vi "test_API_rt.vi"() -> ()   [LabVIEW 2014]
uses:
  MQTT.lvlib
  message acknowledgement.ctl
  MQTT client.lvclass
  QoS levels.ctl
panel:
  in  "connect":bool
  out "subid":i32
  in  "subscribe to":string
  in  "subscribe":bool
  in  "QoS":T1=enum."At least once"
  out "send ID":i32
  out "sub_data":string
  out "sub_topic":string
  out "sub_ID":i32
  out "send failure":T2
  out "send success":T2
  out "QOS Ack":T2
  out "disconnected_message":string
  out "disconnected_code":i32
  out "connCode":i32
  out "connected":string
  in  "stop":bool
  in  "send":bool
  in  "data":string
  in  "topic":string
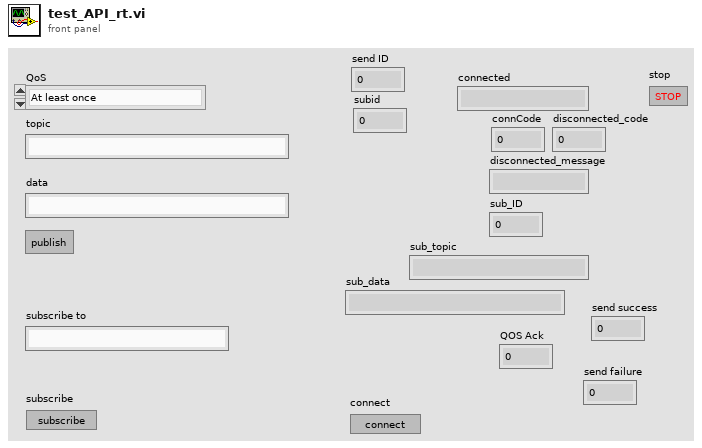
[diagram p1: front panel]
types:
  T1 = typedef "MQTT client.lvclass/QoS levels.ctl" = enum8{"None", "At least once", "Exactly once"}
  T2 = typedef "MQTT client.lvclass/message acknowledgement.ctl" = i32
  T3 = typedef "MQTT.lvlib/events.ctl" = cluster{"subscription":refnum<user-event>, "disconnect":refnum<user-event>, "QoS Ack":refnum<user-event>, "connected":refnum<user-event>, "failed to connect":refnum<user-event>, "send success":refnum<user-event>, "send failure":refnum<user-event>}
  T4 = typedef "MQTT.lvlib/msgAck.ctl" = i32
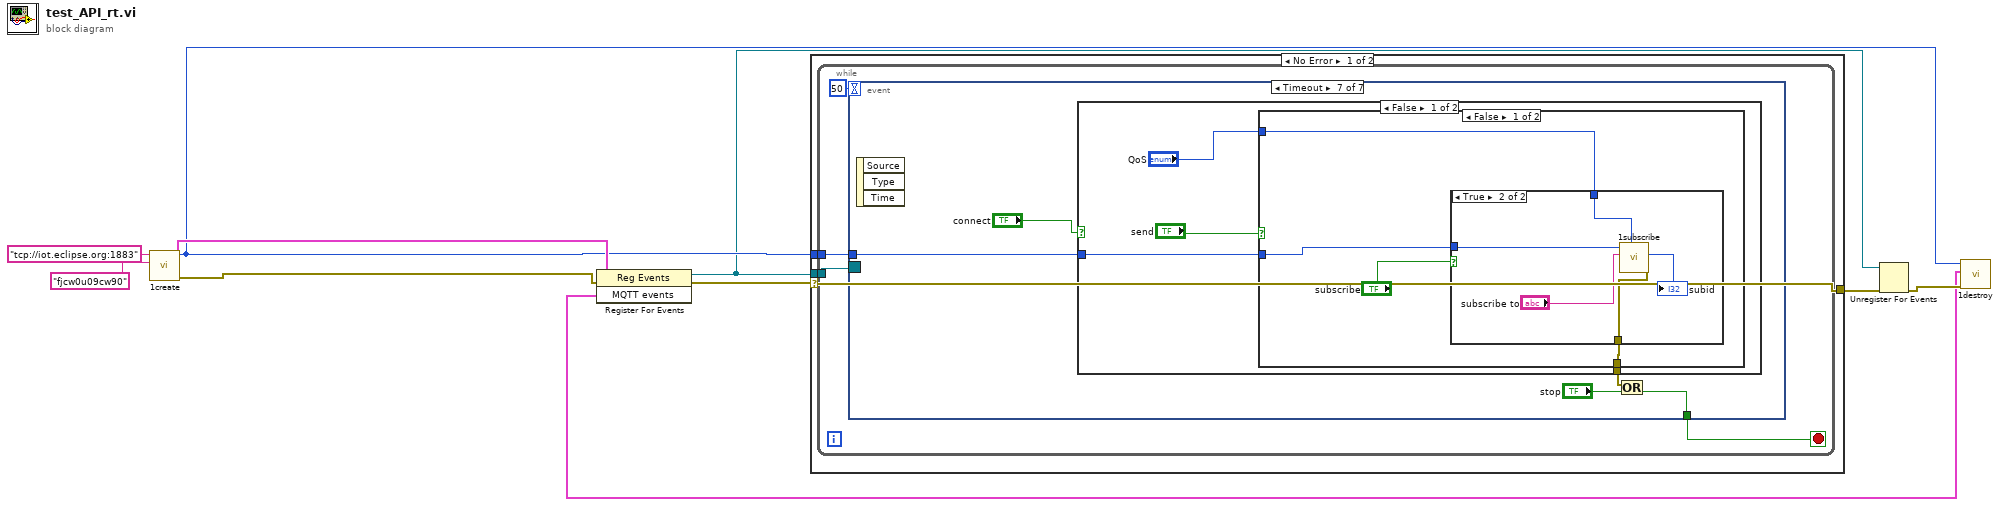
[diagram p0: block diagram]
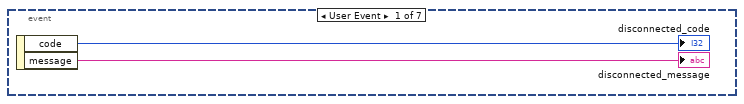
[diagram p2: hidden frame]
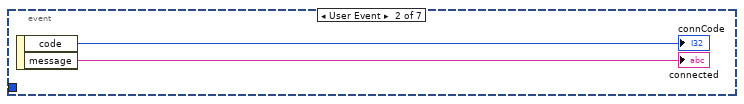
[diagram p3: hidden frame]
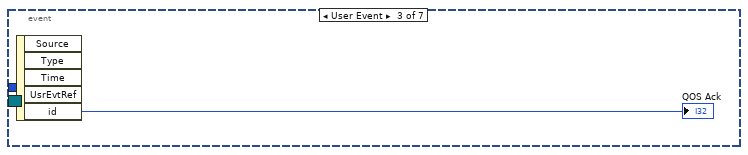
[diagram p4: hidden frame]
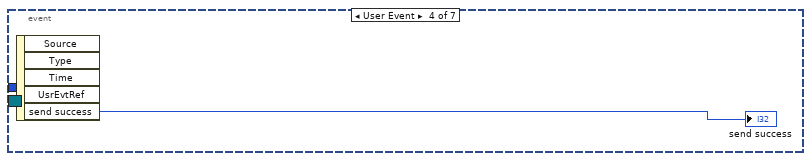
[diagram p5: hidden frame]
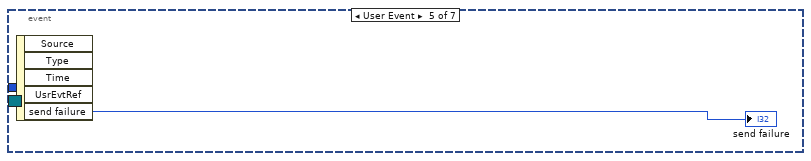
[diagram p6: hidden frame]
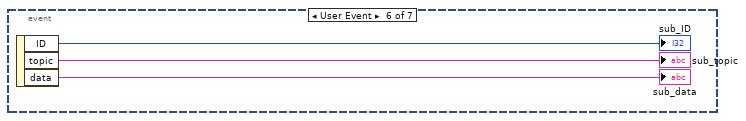
[diagram p7: hidden frame]
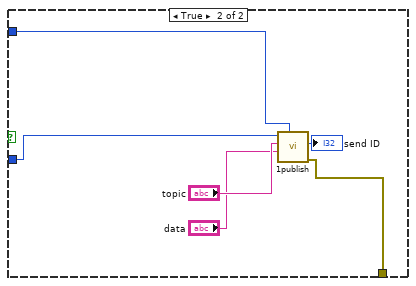
[diagram p9: hidden frame]
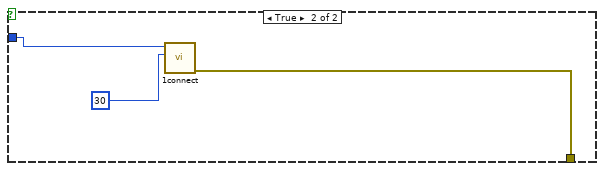
[diagram p10: hidden frame]
diagram:
  n1 = call "1create.vi"("client"="fjcw0u09cw90", "URI"="tcp://iot.eclipse.org:1883") -> ("error out"=w9:errorcluster, "MQTT events"=w3:T3, "MQTT Context"=w2:u64)  [unwired: 7 in]
  n2 = register-events(error in=w9, w3) -> (reference out=w1:refnum<event-registration>, error out=w6:errorcluster)  [unwired: 1 in]
  n3 = case shown="No Error" w6 {
    selector: w6 -> [w10 w54]
    tunnel: w1 -> [w12 _]
    tunnel: [w10 w54] -> w5
    tunnel: w2 -> [w11 _]
    frame No Error {
      n4 = while {
        tunnel: w12 -> [w16]
        tunnel: w11 -> [w15]
        stop <- w14 stop-if-true
        n5 = event shown="[6] Timeout" {
          selector: w16 -> [_ _ _ _ _ _ _]
          dyn-events: _ -> [_ _ _ _ _ _ _]
          timeout: 50 -> [_ _ _ _ _ _ _]
          tunnel: w15 -> [_ _ _ _ _ _ w30]
          tunnel: [_ _ _ _ _ _ w29] -> w14
          event User Event {
            n6 = event-data() -> ("code"=→"disconnected_code":i32, "message"=→"disconnected_message":string)  [unwired: 1 in]
          }
          event User Event {
            n7 = event-data() -> ("code"=→"connCode":i32, "message"=→"connected":string)  [unwired: 1 in]
          }
          event User Event {
            n8 = event-data() -> ("id"=→"QOS Ack":T4)  [unwired: 1 in, 4 out]
          }
          event User Event {
            n9 = event-data() -> ("send success"=→"send success":T4)  [unwired: 1 in, 4 out]
          }
          event User Event {
            n10 = event-data() -> ("send failure"=→"send failure":T4)  [unwired: 1 in, 4 out]
          }
          event User Event {
            n11 = event-data() -> ("ID"=→"sub_ID":i32, "topic"=→"sub_topic":string, "data"=→"sub_data":string)  [unwired: 1 in]
          }
          event Timeout {
            n12 = event-data() -> ()  [unwired: 1 in, 3 out]
            n13 = case shown="False" "connect" {
              tunnel: w30 -> [w34 w52]
              tunnel: [w32 w51] -> w28
              frame False {
                n14 = case shown="False" "send" {
                  tunnel: "QoS" -> [w39 w46]
                  tunnel: w34 -> [w37 w47]
                  tunnel: [w36 w45] -> w32
                  frame False {
                    n15 = case shown="True" "subscribe" {
                      tunnel: w39 -> [_ w42]
                      tunnel: w37 -> [_ w41]
                      tunnel: [_ w40] -> w36
                      frame False {
                      }
                      frame True {
                        n16 = call "1subscribe.vi"("QoS"=w42, "topic"="subscribe to", "MQTT Context in"=w41) -> ("error out"=w40:errorcluster, "send ID"=→"subid":i32)  [unwired: 6 in, 1 out]
                      }
                    }
                  }
                  frame True {
                    n17 = call "1publish.vi"("QoS"=w46, "data"="data", "topic"="topic", "MQTT Context in"=w47) -> ("error out"=w45:errorcluster, "send ID"=→"send ID":i32)  [unwired: 5 in, 1 out]
                  }
                }
              }
              frame True {
                n18 = call "1connect.vi"("timeout"=30, "MQTT Context in"=w52) -> ("error out"=w51:errorcluster)  [unwired: 8 in, 1 out]
              }
            }
            n19 = Or(x=w28, y="stop") -> (x .or. y?=w29:bool)
          }
        }
      }
    }
    frame Error {
    }
  }
  n20 = Unregister For Events(event registration refnum=w1, error in=w5) -> (error out=w4:errorcluster)
  n21 = call "1destroy.vi"("error in)"=w4, "MQTT events"=w3, "MQTT Context"=w2) -> ()  [unwired: 8 in, 1 out]
